vi "Do Mux Selection.vi"(6 "MUX Selection":T1, 8 "error in (no error)":errorcluster, 9 "Input Index":i32, 10 "Output Index":i32, 11 "MuxPanel in":refnum<class "MuxPanel.lvclass">) -> (0 "error out":errorcluster, 3 "MuxPanel out":refnum<class "MuxPanel.lvclass">)   [LabVIEW 2022 SP3, in "TouchControl.lvlib" / "MuxPanel.lvclass"]
uses:
  MuxPanel.lvclass
  MUX Selection.ctl
  MuxPanel.lvclass/MuxPanel.ctl
  <vilib>/httpClient/LabVIEWHTTPClient.lvlib
  TouchControl.lvlib
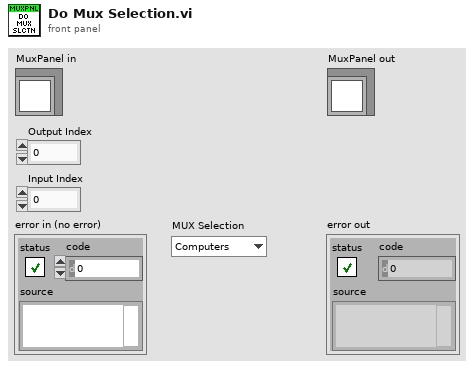
[diagram p1: front panel]
types:
  T1 = typedef "TouchControl.lvlib/MUX Selection.ctl" = enum16{"Computers", "Others"}
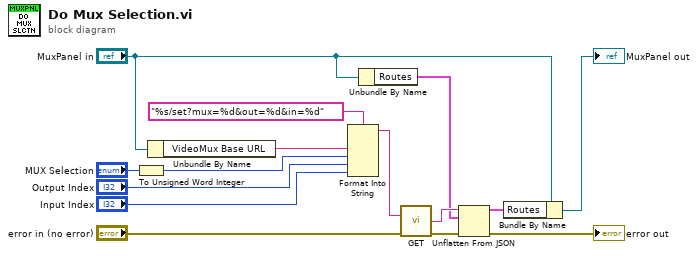
[diagram p0: block diagram]
diagram:
  n1 = To Unsigned Word Integer(number="MUX Selection") -> (unsigned 16bit integer=w12:u16)
  n2 = Unbundle By Name("MuxPanel in") -> ("VideoMux Base URL"=w13:string)
  n3 = Format Into String(format string="%s/set?mux=%d&out=%d&in=%d", w13, w12, "Output Index", "Input Index") -> (resulting string=w9:string)  [unwired: 2 in, 1 out]
  n4 = Unbundle By Name("MuxPanel in") -> ("Routes"=w5:cluster{"Mux Route":i32[]}[])
  n5 = call <vilib>:"GET.vi"("url"=w9, "error in (no error)"="error in (no error)") -> ("body"=w6:string, "error out"=w7:errorcluster)  [unwired: 10 in, 2 out]
  n6 = Unflatten From JSON(JSON string=w6, type and defaults=w5, error in (no error)=w7) -> (value=w4:cluster{"Mux Route":i32[]}[], error out=→"error out":errorcluster)  [unwired: 4 in]
  n7 = Bundle By Name(cluster="MuxPanel in", "Routes"=w4) -> (→"MuxPanel out":refnum<class "MuxPanel.lvclass">)
